vi "SweepSetupOG.vi"(0 "VISA IN":refnum<visa-resource-name>, 5 "error in":errorcluster) -> (14 "VISA Out":refnum<visa-resource-name>, 19 "error out":errorcluster)   [LabVIEW 2018, in "PNA-X.lvlib"]
uses:
  PNA-X.lvlib
panel:
  in  "Sweep Time ON/OFF":bool
  in  "Sweep Mode(ALL or NONE)":string(combo)="NONE"
  in  "Dwell Time(sec)":dbl
  in  "Source Frq. Mode":string(combo)="STEPped"
  in  "Sweep Type":string(combo)="LINear"
  in  "Channel":i32=1
  in  "Npoints":dbl=1.0
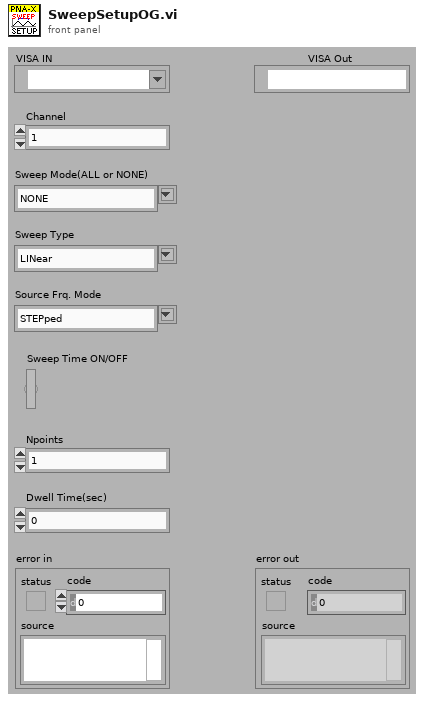
[diagram p1: front panel]
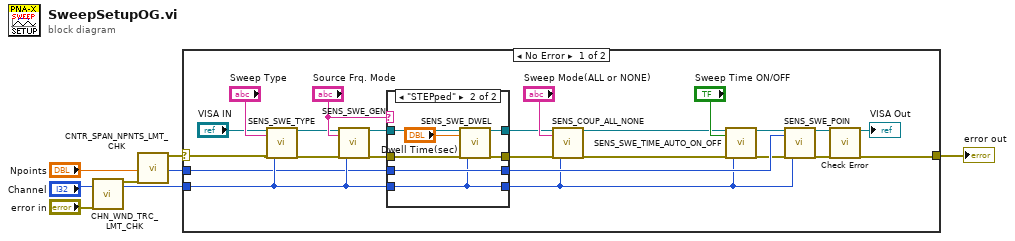
[diagram p0: block diagram]
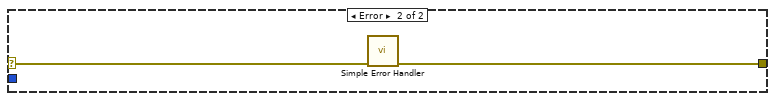
[diagram p3: hidden frame]
diagram:
  n1 = call "CHN_WND_TRC_LMT_CHK.vi"("Channel"="Channel", "error in"="error in") -> ("error out"=w8:errorcluster, "Channel"=w2:i32)  [unwired: 13 in, 3 out]
  n2 = call "CNTR_SPAN_NPNTS_LMT_CHK.vi"("Npoints"="Npoints", "error in"=w8) -> ("error out"=w3:errorcluster, "Npoints"=w1:i32)  [unwired: 14 in, 2 out]
  n3 = case shown="No Error" w3 {
    selector: w3 -> [w26 w45]
    tunnel: [w32 w44] -> w5
    tunnel: w2 -> [w28 _]
    tunnel: w1 -> [w25 _]
    frame No Error {
      n4 = call "SENS_SWE_TYPE.vi"("VISA IN"="VISA IN", "Sweep Type"="Sweep Type", "error in"=w26, "Channel"=w28) -> ("VISA Out"=w18:refnum<visa-resource-name>, "error out"=w17:errorcluster)  [unwired: 14 in]
      n5 = call "SENS_SWE_GEN.vi"("VISA IN"=w18, "Source Frq. Mode"="Source Frq. Mode", "error in"=w17, "Channel"=w28) -> ("VISA Out"=w16:refnum<visa-resource-name>, "error out"=w15:errorcluster)  [unwired: 14 in]
      n6 = case shown="\"STEPped\"" "Source Frq. Mode" {
        tunnel: w28 -> [w35 w37]
        tunnel: w25 -> [w36 w43]
        tunnel: [w36 w43] -> w24
        tunnel: [w35 w37] -> w23
        tunnel: w15 -> [w33 w42]
        tunnel: [w33 w41] -> w13
        tunnel: w16 -> [w34 w40]
        tunnel: [w34 w39] -> w14
        frame Default {
        }
        frame "STEPped" {
          n7 = call "SENS_SWE_DWEL.vi"("VISA IN"=w40, "Dwell Time(sec)"="Dwell Time(sec)", "error in"=w42, "Channel"=w37) -> ("VISA Out"=w39:refnum<visa-resource-name>, "error out"=w41:errorcluster)  [unwired: 14 in]
        }
      }
      n8 = call "SENS_COUP_ALL_NONE.vi"("VISA IN"=w14, "Sweep Mode(ALL or NONE)"="Sweep Mode(ALL or NONE)", "error in"=w13, "Channel"=w23) -> ("VISA Out"=w12:refnum<visa-resource-name>, "error out"=w11:errorcluster)  [unwired: 14 in]
      n9 = call "SENS_SWE_TIME_AUTO_ON_OFF.vi"("VISA IN"=w12, "Sweep Time ON/OFF"="Sweep Time ON/OFF", "error in"=w11, "Channel"=w23) -> ("VISA Out"=w10:refnum<visa-resource-name>, "error out"=w9:errorcluster)  [unwired: 14 in]
      n10 = call "SENS_SWE_POIN.vi"("VISA IN"=w10, "Sweep Points"=w24, "error in"=w9, "Channel"=w23) -> ("VISA Out"=w19:refnum<visa-resource-name>, "error out"=w20:errorcluster)  [unwired: 14 in]
      n11 = call "Check Error.vi"("VISA Resource Name"=w19, "error in (no error)"=w20) -> ("dup VISA session"=→"VISA Out":refnum<visa-resource-name>, "error out"=w32:errorcluster)  [unwired: 16 in]
    }
    frame Error {
      n12 = call <vilib>:"Simple Error Handler.vi"("error in (no error)"=w45) -> ("error out"=w44:errorcluster)  [unwired: 4 in, 4 out]
    }
  }
  "error out" <- w5
